vi "odor temporal control panel with graphing.vi"() -> ()   [LabVIEW 2013]
uses:
  <vilib>/DAQmx/write.llb/DAQmx Write (Digital Bool 1Line 1Point).vi
  Image Aquisition - Labview/Image Recorder/experiment state global.vi
  <vilib>/DAQmx/miscellaneous.llb/DAQmx Fill In Error Info.vi
panel:
  in  "meas to display":u16(ring) items=["ms timer", "air_sp", "odor1_sp", "odor2_sp", "co2_sp", "air_fr", "odor1_fr", "odor2_fr", "co2_fr", "pid_reading"]
  out "measurements":cluster{"X":dbl, "Y":dbl}[](graph)
  in  "reset":bool
  in  "direct control of digital lines":bool
  in  "digital controls":T1
  out "flow rates":T2 {"pid reading" format="%0.2f"}
  out "setpoints":T3={"Air "=1.0, "odor1"=0.0, "odor2"=0.0, "co2"=0.0}
  in  "gradient settings":T4={"air settings"={"enabled"=TRUE, "temporal ramp type"=enum."Square", "period(s)"=1200.0, "high limit"=4.0, "low limit"=1.0, "duty cycle (sq wave)"=50.0, "phase shift (deg)"=0.0, "value to output when disabled"=1.0}, "odor1 settings"={"enabled"=FALSE, "temporal ramp type"=enum."Sine", "period(s)"=120.0, "high limit"=100.0, "low limit"=0.0, "duty cycle (sq wave)"=50.0, "phase shift (deg)"=0.0, "value to output when disabled"=0.0}, "odor2 settings"={"enabled"=FALSE, "temporal ramp type"=enum."Sine", "period(s)"=120.0, "high limit"=100.0, "low limit"=0.0, "duty cycle (sq wave)"=50.0, "phase shift (deg)"=0.0, "value to output when disabled"=0.0}, "co2 settings"={"enabled"=TRUE, "temporal ramp type"=enum."Triangle", "period(s)"=200.0, "high limit"=200.0, "low limit"=0.0, "duty cycle (sq wave)"=50.0, "phase shift (deg)"=-90.0, "value to output when disabled"=0.0}} {"co2 settings"."value to output when disabled" min=0.0; "co2 settings"."low limit" format="%#_6p"; "odor2 settings"."value to output when disabled" max=100.0; "odor2 settings"."low limit" format="%#_6p"; "odor2 settings"."high limit" max=100.0; "odor1 settings"."value to output when disabled" max=100.0; "odor1 settings"."low limit" format="%#_6p"; "odor1 settings"."high limit" max=100.0; "air settings"."value to output when disabled" max=100.0; "air settings"."low limit" format="%#_6p"; "air settings"."high limit" max=100.0}
  in  "Sync Gradient To Image Aquisition":bool=TRUE
  in  "enable gradient":bool
  in  "restart gradient":bool
  in  "update period (ms)":u32=100
  in  "stop":bool
  out "error out":errorcluster
  # "restarting gradient also enables output"
  # "maximum amplitude is 100"
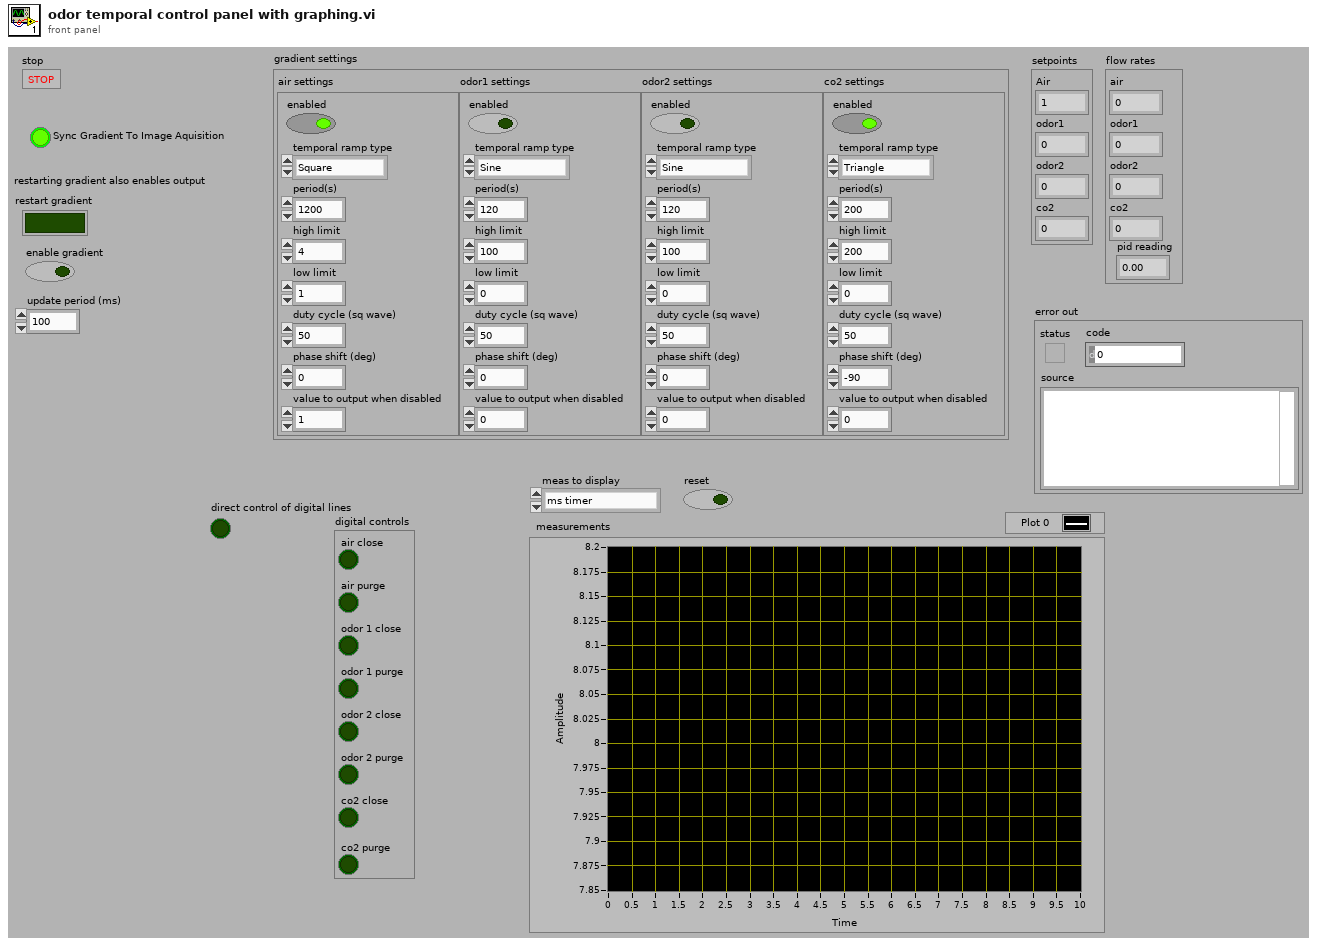
[diagram p1: front panel]
types:
  T1 = cluster{"air close":bool, "air purge":bool, "odor 1 close":bool, "odor 1 purge":bool, "odor 2 close":bool, "odor 2 purge":bool, "co2 close":bool, "co2 purge":bool}
  T2 = cluster{"air":dbl, "odor1":dbl, "odor2":dbl, "co2":dbl, "pid reading":dbl}
  T3 = cluster{"Air ":dbl, "odor1":dbl, "odor2":dbl, "co2":dbl}
  T4 = cluster{"air settings":cluster{"enabled":bool, "temporal ramp type":enum16{"Sine", "Triangle", "Sawtooth", "Square", "Exponential"}, "period(s)":dbl, "high limit":dbl, "low limit":dbl, "duty cycle (sq wave)":dbl, "phase shift (deg)":dbl, "value to output when disabled":dbl}, "odor1 settings":cluster{"enabled":bool, "temporal ramp type":enum16{"Sine", "Triangle", "Sawtooth", "Square", "Exponential"}, "period(s)":dbl, "high limit":dbl, "low limit":dbl, "duty cycle (sq wave)":dbl, "phase shift (deg)":dbl, "value to output when disabled":dbl}, "odor2 settings":cluster{"enabled":bool, "temporal ramp type":enum16{"Sine", "Triangle", "Sawtooth", "Square", "Exponential"}, "period(s)":dbl, "high limit":dbl, "low limit":dbl, "duty cycle (sq wave)":dbl, "phase shift (deg)":dbl, "value to output when disabled":dbl}, "co2 settings":cluster{"enabled":bool, "temporal ramp type":enum16{"Sine", "Triangle", "Sawtooth", "Square", "Exponential"}, "period(s)":dbl, "high limit":dbl, "low limit":dbl, "duty cycle (sq wave)":dbl, "phase shift (deg)":dbl, "value to output when disabled":dbl}}
  T5 = cluster{"millisecond timer value":u32, "setpoints ":cluster{"Air ":dbl, "odor1":dbl, "odor2":dbl, "co2":dbl}, "flow rates":cluster{"air":dbl, "odor1":dbl, "odor2":dbl, "co2":dbl, "pid reading":dbl}}
  T6 = cluster{"analog output channels":cluster{"air ao":refnum<k21>, "odor 1 ao":refnum<k21>, "odor 2 ao":refnum<k21>, "co2 ao":refnum<k21>}, "analog input channels":cluster{"air ai":refnum<k21>, "odor 1 ai":refnum<k21>, "odor 2 ai":refnum<k21>, "co2 ai":refnum<k21>, "pid sensor 1 ai":refnum<k21>, "pid sensor 2 ai":refnum<k21>}, "digital control lines":cluster{"air close":refnum<k21>, "air purge":refnum<k21>, "odor 1 close":refnum<k21>, "odor 1 purge":refnum<k21>, "odor 2 close":refnum<k21>, "odor 2 purge":refnum<k21>, "co2 close":refnum<k21>, "co2 purge":refnum<k21>}}
  T7 = cluster{"experiment started":bool, "experiment ended":bool, "experiment start time":u32}
  T8 = cluster{"air close":refnum<k21>, "air purge":refnum<k21>, "odor 1 close":refnum<k21>, "odor 1 purge":refnum<k21>, "odor 2 close":refnum<k21>, "odor 2 purge":refnum<k21>, "co2 close":refnum<k21>, "co2 purge":refnum<k21>}
  T9 = cluster{"millisecond timer value":u32, "setpoints ":cluster{"Air ":dbl, "odor1":dbl, "odor2":dbl, "co2":dbl}, "flow rates":cluster{"air":dbl, "odor1":dbl, "odor2":dbl, "co2":dbl, "pid reading":dbl}}[]
  T10 = cluster{"data directory":path, "file stub":string}
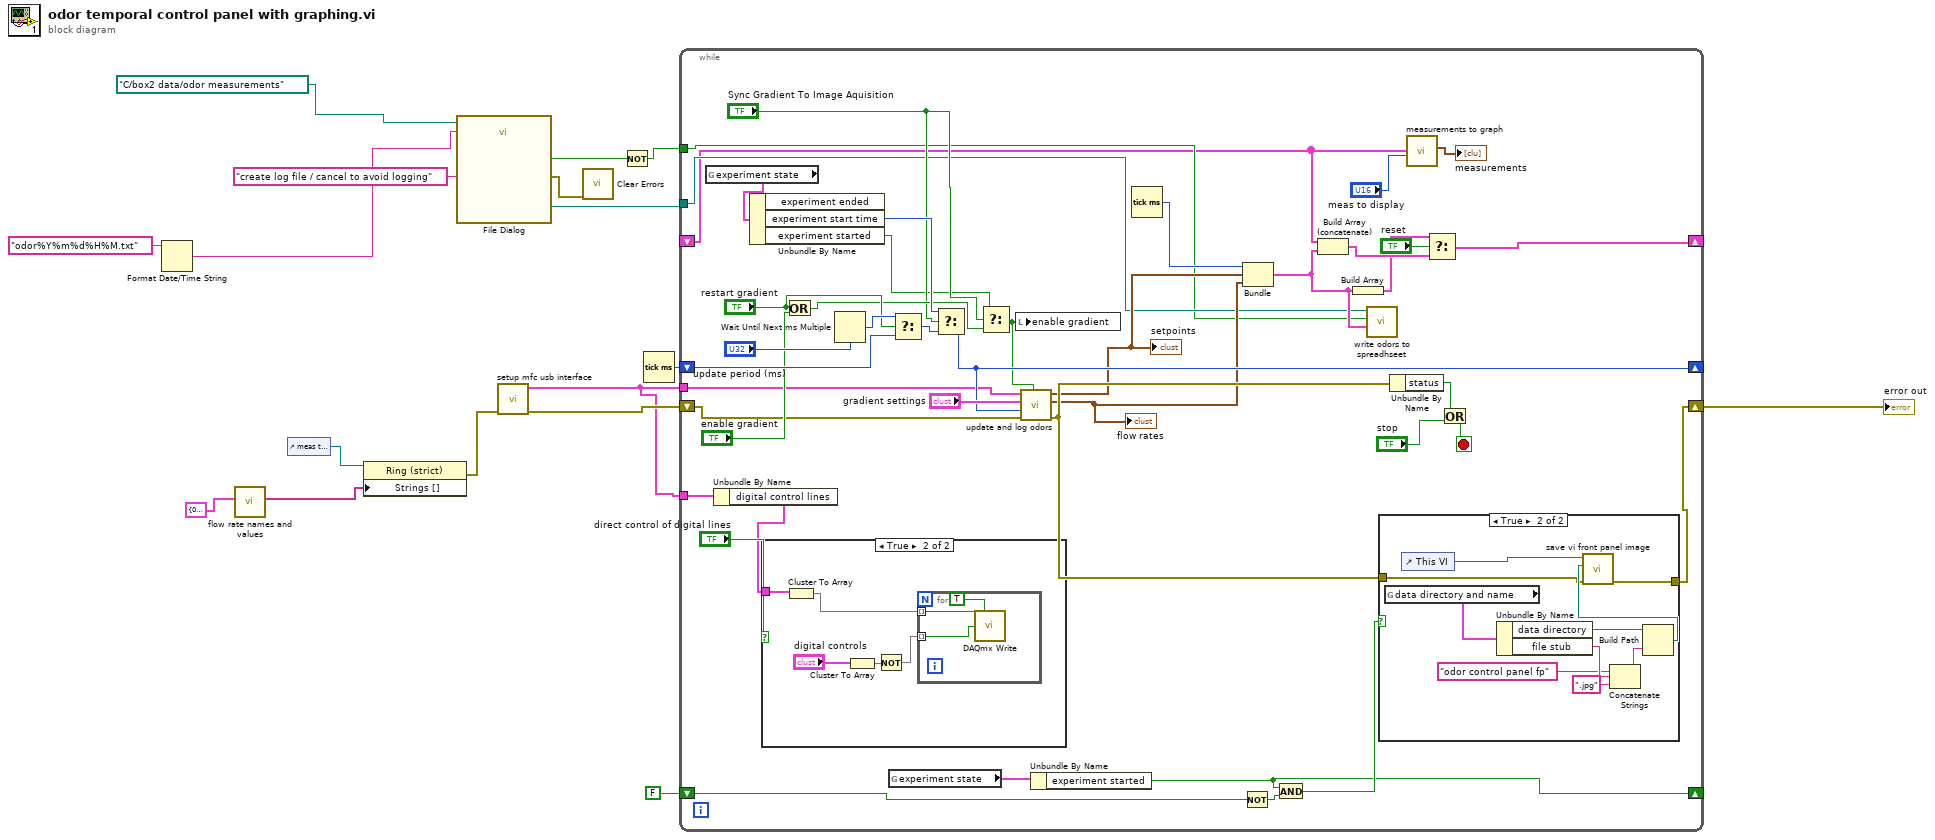
[diagram p0: block diagram]
diagram:
  n1 = Format Date/Time String(time format string (%c)="odor%Y%m%d%H%M.txt") -> (date/time string=w2:string)  [unwired: 2 in]
  n2 = call "flow rate names and values.vi"("measurements"=T5 {"millisecond timer value"=0, "setpoints "={"Air "=0.0, "odor1"=0.0, "odor2"=0.0, "co2"=0.0}, "flow rates"={"air"=0.0, "odor1"=0.0, "odor2"=0.0, "co2"=0.0, "pid reading"=0.0}} ("output cluster")) -> ("names"=w5:string[])  [unwired: 9 in, 1 out]
  n3 = control-ref of="meas to display"() -> (w8:refnum<vi>)
  n4 = property class="Ring (strict)"(reference=w8, "Strings []"=w5) -> (error out=w6:errorcluster)  [unwired: 1 in, 1 out]
  n5 = call "File Dialog"("start path"=path "C:/box2 data/odor measurements", "prompt"="create log file / cancel to avoid logging", "default name"=w2) -> ("selected path"=w10:path, "cancelled"=w9:bool, "error out"=w4:errorcluster)  [unwired: 9 in, 1 out]
  n6 = call "setup mfc usb interface.vi"("error in"=w6) -> ("error out"=w16:errorcluster, "daqmx tasks"=w13:T6)  [unwired: 9 in]
  n7 = call <vilib>:"Clear Errors.vi"("error in (no error)"=w4) -> ()  [unwired: 6 in, 1 out]
  n8 = Not(x=w9) -> (.not. x?=w3:bool)
  n9 = Tick Count (ms)() -> (millisecond timer value=w17:u32)
  n10 = while {
    shift-right: [w40] -> w15
    shift-left: w16 -> [w37]
    shift-right: [w38] -> _
    shift-left: w17 -> [w56]
    tunnel: w13 -> [w35]
    shift-right: [w42] -> _
    shift-left: FALSE ("experiment started") -> [w41]
    tunnel: w13 -> [w33]
    shift-right: [w27] -> _
    shift-left: _ -> [w20]
    tunnel: w10 -> [w22]
    tunnel: w3 -> [w21]
    stop <- w59 stop-if-true
    n11 = global read "experiment state global.vi" "experiment state"() -> (w51:T7)
    n12 = Unbundle By Name(w33) -> ("digital control lines"=w31:T8)
    n13 = Unbundle By Name(w51) -> ("experiment start time"=w50:u32, "experiment started"=w46:bool)  [unwired: 1 out]
    n14 = case shown="True" "direct control of digital lines" {
      tunnel: w31 -> [_ w63]
      frame False {
      }
      frame True {
        n15 = Cluster To Array(cluster=w63) -> (array=w61:refnum<k21>[])
        n16 = Cluster To Array(cluster="digital controls") -> (array=w62:bool[])
        n17 = Not(x=w62) -> (.not. x?=w60:bool[])
        n18 = for {
          tunnel: w61 -> [w67] mode=indexing
          tunnel: w60 -> [w66] mode=indexing
          n19 = call-poly <vilib>:"DAQmx Write.vi"("task/channels in"=w67, "auto start"=TRUE, "data"=w66) -> ()  [unwired: 10 in, 3 out]
        }
      }
    }
    n20 = Or(x="restart gradient", y="enable gradient") -> (x .or. y?=w49:bool)
    n21 = Wait Until Next ms Multiple(millisecond multiple="update period (ms)") -> (millisecond timer value=w55:u32)
    n22 = global read "experiment state global.vi" "experiment state"() -> (w43:T7)
    n23 = Select(t=w55, s="restart gradient", f=w56) -> (s? t:f=w52:u32)
    n24 = Select(t=w50, s="Sync Gradient To Image Aquisition", f=w52) -> (s? t:f=w38:u32)
    n25 = Select(t=w46, s="Sync Gradient To Image Aquisition", f=w49) -> (s? t:f=w36:bool)
    n26 = local write "enable gradient"(w36) -> ()
    n27 = call "update and log odors.vi"("global enable"=w36, "error in"=w37, "t0"=w38, "gradient settings"="gradient settings", "daqmx tasks"=w35) -> ("error out"=w34:errorcluster, "flow rates"=w29:T2, "setpoints"=w30:T3)  [unwired: 4 in]
    "setpoints" <- w30
    "flow rates" <- w29
    n28 = Unbundle By Name(w43) -> ("experiment started"=w42:bool)
    n29 = Tick Count (ms)() -> (millisecond timer value=w28:u32)
    n30 = Not(x=w41) -> (.not. x?=w45:bool)
    n31 = Bundle("millisecond timer value"=w28, "setpoints"=w30, "flow rates"=w29) -> (w23:T5)  [unwired: 1 in]
    n32 = And(x=w42, y=w45) -> (x .and. y?=w44:bool)
    n33 = Build Array (concatenate)(w20, w23) -> (w26:T9)
    n34 = Build Array(w23) -> (w25:T9)
    n35 = call "write odors to spreadhseet.vi"("measurements"=w23, "write odors?"=w21, "file path"=w22) -> ()  [unwired: 9 in]
    n36 = case shown="True" w44 {
      tunnel: [w68 w70] -> w40
      tunnel: w34 -> [w68 w69]
      frame False {
      }
      frame True {
        n37 = global read "experiment state global.vi" "data directory and name"() -> (w77:T10)
        n38 = control-ref of="This VI"() -> (w78:refnum<vi>)
        n39 = Unbundle By Name(w77) -> ("data directory"=w76:path, "file stub"=w75:string)
        n40 = Concatenate Strings("odor control panel fp" ("string"), w75, ".jpg" ("string")) -> (w72:string)
        n41 = Build Path(base path=w76, name or relative path=w72) -> (appended path=w71:path)
        n42 = call "save vi front panel image.vi"("error in (no error)"=w69, "path to JPEG file"=w71, "This VI"=w78) -> ("error out"=w70:errorcluster)  [unwired: 8 in]
      }
    }
    n43 = Unbundle By Name(w34) -> ("status"=w53:bool)
    n44 = call "measurements to graph.vi"("index"="meas to display", "measurements"=w20) -> ("graph values"=→"measurements":cluster{dbl, "pid reading":dbl}[])  [unwired: 9 in]
    n45 = Select(t=w25, s="reset", f=w26) -> (s? t:f=w27:T9)
    n46 = Or(x=w53, y="stop") -> (x .or. y?=w59:bool)
  }
  "error out" <- w15
